vi "(SubVI)Mode Event.vi"(7 "Function (Gen)":T2=enum."Gen Event", 8 "error in (no error)":errorcluster caption="에러 입력(에러 없음)", 11 "Event Type":T1) -> (0 "error out":errorcluster caption="에러 출력", 3 "Mode Event":refnum<user-event>)   [LabVIEW 2020]
uses:
  Controls/(Ctrl)Mode Event_Event Type.ctl
  Controls/(Ctrl)Mode Event_FGV Function.ctl
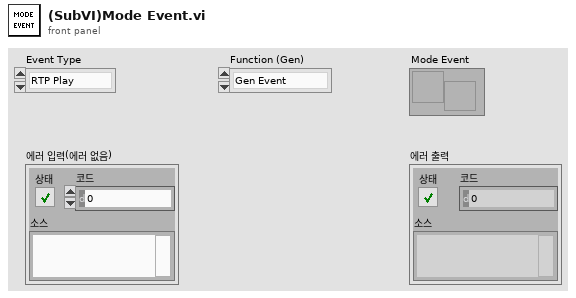
[diagram p1: front panel]
types:
  T1 = typedef "(Ctrl)Mode Event_Event Type.ctl" = enum16{"RTP Play", "RTP Stop", "Scope Start", "Scope Stop"}
  T2 = typedef "(Ctrl)Mode Event_FGV Function.ctl" = enum16{"Init", "Get Event Ref", "Gen Event", "Destroy"}
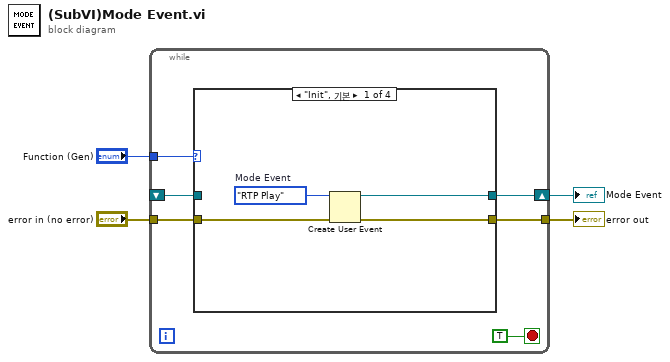
[diagram p0: block diagram]
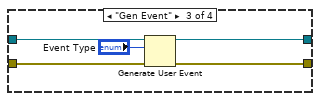
[diagram p3: hidden frame]
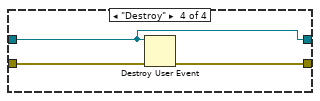
[diagram p4: hidden frame]
diagram:
  n1 = while {
    tunnel: "Function (Gen)" -> [w9]
    tunnel: [w8] -> w3
    shift-right: [w7] -> w1
    shift-left: _ -> [w6]
    tunnel: "error in (no error)" -> [w5]
    stop <- TRUE stop-if-true
    n2 = case shown="\"Init\", 기본" w9 {
      tunnel: [w13 w15 w20 w23] -> w8
      tunnel: [w12 w16 w18 w22] -> w7
      tunnel: w6 -> [_ w16 w19 w22]
      tunnel: w5 -> [w14 w15 w21 w24]
      frame "Init", Default {
        w11 = (Ctrl)Mode_Event_Event_Type."RTP Play"  # Mode Event
        n3 = Create User Event(user event datatype=w11, error in=w14) -> (user event=w12:refnum<user-event>, error out=w13:errorcluster)
      }
      frame "Get Event Ref" {
      }
      frame "Gen Event" {
        n4 = Generate User Event(user event=w19, event data cluster="Event Type", error in=w21) -> (user event out=w18:refnum<user-event>, error out=w20:errorcluster)  [unwired: 1 in]
      }
      frame "Destroy" {
        n5 = Destroy User Event(user event=w22, error in=w24) -> (error out=w23:errorcluster)
      }
    }
  }
  "error out" <- w3
  "Mode Event" <- w1
